vi "Get Buffer.vi"(11 "AI Current DAQmx Cont CFG in":refnum<class "AI Current DAQmx Cont CFG.lvclass">) -> (2 "Buffer Lossless DBL":refnum<class "Buffer Lossless DBL.lvclass">, 3 "AI Current DAQmx Cont CFG out":refnum<class "AI Current DAQmx Cont CFG.lvclass">)   [LabVIEW 2024, in "AI Current DAQmx Cont CFG.lvclass"]
uses:
  AI Current DAQmx Cont CFG.lvclass
  AI Current DAQmx Cont CFG.lvclass/AI Current DAQmx Cont CFG.ctl
  Buffers/Buffer Lossless DBL/Buffer Lossless DBL.lvclass
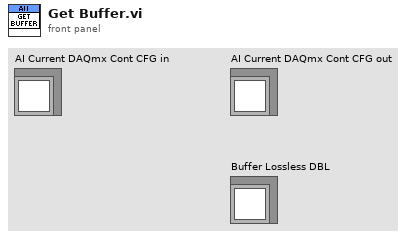
[diagram p1: front panel]
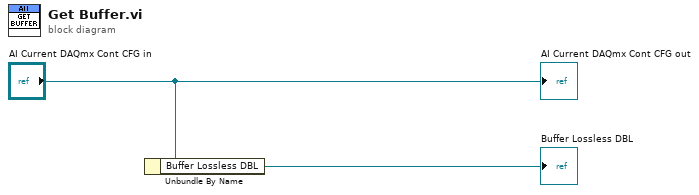
[diagram p0: block diagram]
diagram:
  n1 = Unbundle By Name("AI Current DAQmx Cont CFG in") -> ("Buffer Lossless DBL"=→"Buffer Lossless DBL":refnum<class "Buffer Lossless DBL.lvclass">)
  "AI Current DAQmx Cont CFG out" <- "AI Current DAQmx Cont CFG in"
